vi "daq_intergration_v5.vi"() -> ()   [LabVIEW 2019]
uses:
  <vilib>/DAQmx/write.llb/DAQmx Write (Digital Bool 1Line 1Point).vi
  <vilib>/DAQmx/write.llb/DAQmx Write (Analog 1D DBL 1Chan NSamp).vi
  <vilib>/DAQmx/write.llb/DAQmx Write (Analog DBL 1Chan 1Samp).vi
  <vilib>/DAQmx/read.llb/DAQmx Read (Analog 1D Wfm NChan NSamp).vi
  <vilib>/DAQmx/create/channels.llb/DAQmx Create Channel (DO-Digital Output).vi
  <vilib>/DAQmx/miscellaneous.llb/DAQmx Fill In Error Info.vi
  <vilib>/DAQmx/create/channels.llb/DAQmx Create Channel (AI-Voltage-Basic).vi
  <vilib>/DAQmx/configure/timing.llb/DAQmx Timing (Sample Clock).vi
  <vilib>/DAQmx/configure/task.llb/DAQmx Configure Logging (TDMS).vi
  <vilib>/DAQmx/create/channels.llb/DAQmx Create Channel (AO-Voltage-Basic).vi
  <vilib>/measure/NI_MABase.lvlib
panel:
  in  "amplitude 3":dbl=2.5 caption="强刺激幅值" format="%0.2p"
  in  "强刺激频率":dbl=10.0 format="%#_13g"
  in  "低电平时间":dbl=15.0
  in  "高电平时间":dbl=10.0
  in  "physical channels 4":tag="Dev2/port0/line2" caption="行为视频输出通道"
  in  "行为视频":bool
  in  "刺激间隔下限(s)":dbl=3.0
  in  "刺激间隔上限":dbl=5.0
  in  "lines 2":tag="Dev2/port0/line1" caption="刺激事件通道"
  in  "frequency 2":dbl=10.0 caption="弱刺激频率" format="%0.2p"
  in  "amplitude 2":dbl=1.5 caption="弱刺激幅值" format="%0.2p"
  in  "amplitude":dbl=0.5 caption="超弱刺激幅值" format="%0.2p"
  in  "frequency":dbl=10.0 caption="超弱刺激频率" format="%0.2p"
  in  "physical channels 3":tag="Dev2/ao1" caption="胡须刺激通道"
  in  "胡须刺激":bool
  in  "data":dbl=2.0 caption="光源电压" format="%0.2f"
  in  "LED 光源":bool
  in  "physical channels 2":tag="Dev2/ao0" caption="LED通道"
  in  "lines":tag="Dev2/port0/line0" caption="事件通道"
  in  "?":bool
  in  "logging mode":i32(ring)=10231 caption="记录模式" items=["关"=10231, "记录"=15844, "记录并读取"=15842]
  in  "samples per channel":i32=1000 caption="每通道采样"
  in  "physical channels":tag="Dev2/ai0:3" caption="输入通道"
  in  "file path":path caption="文件路径"
  in  "停止":bool
  out "波形图":waveform(dbl)[](graph)
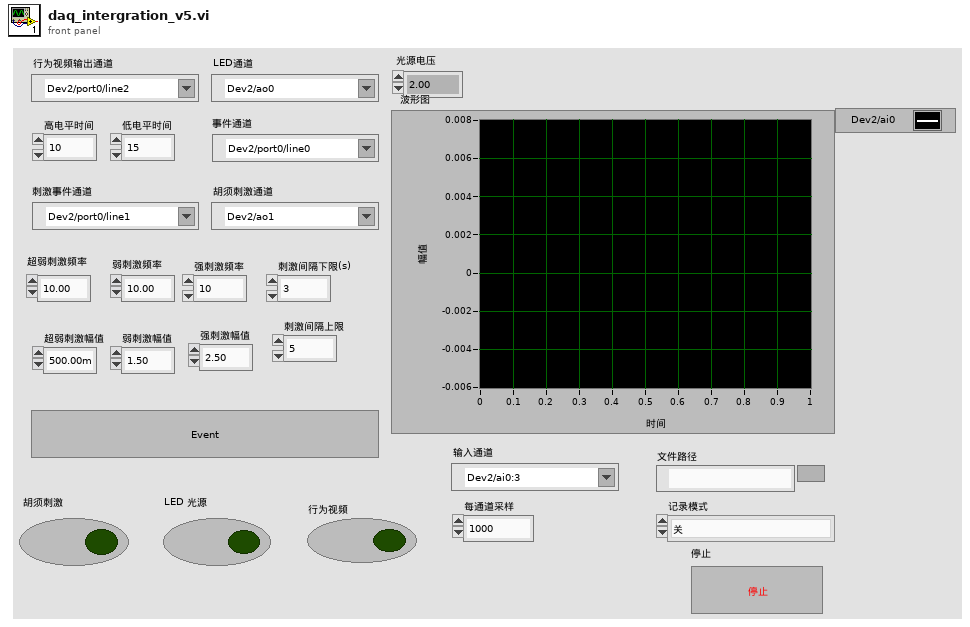
[diagram p1: front panel]
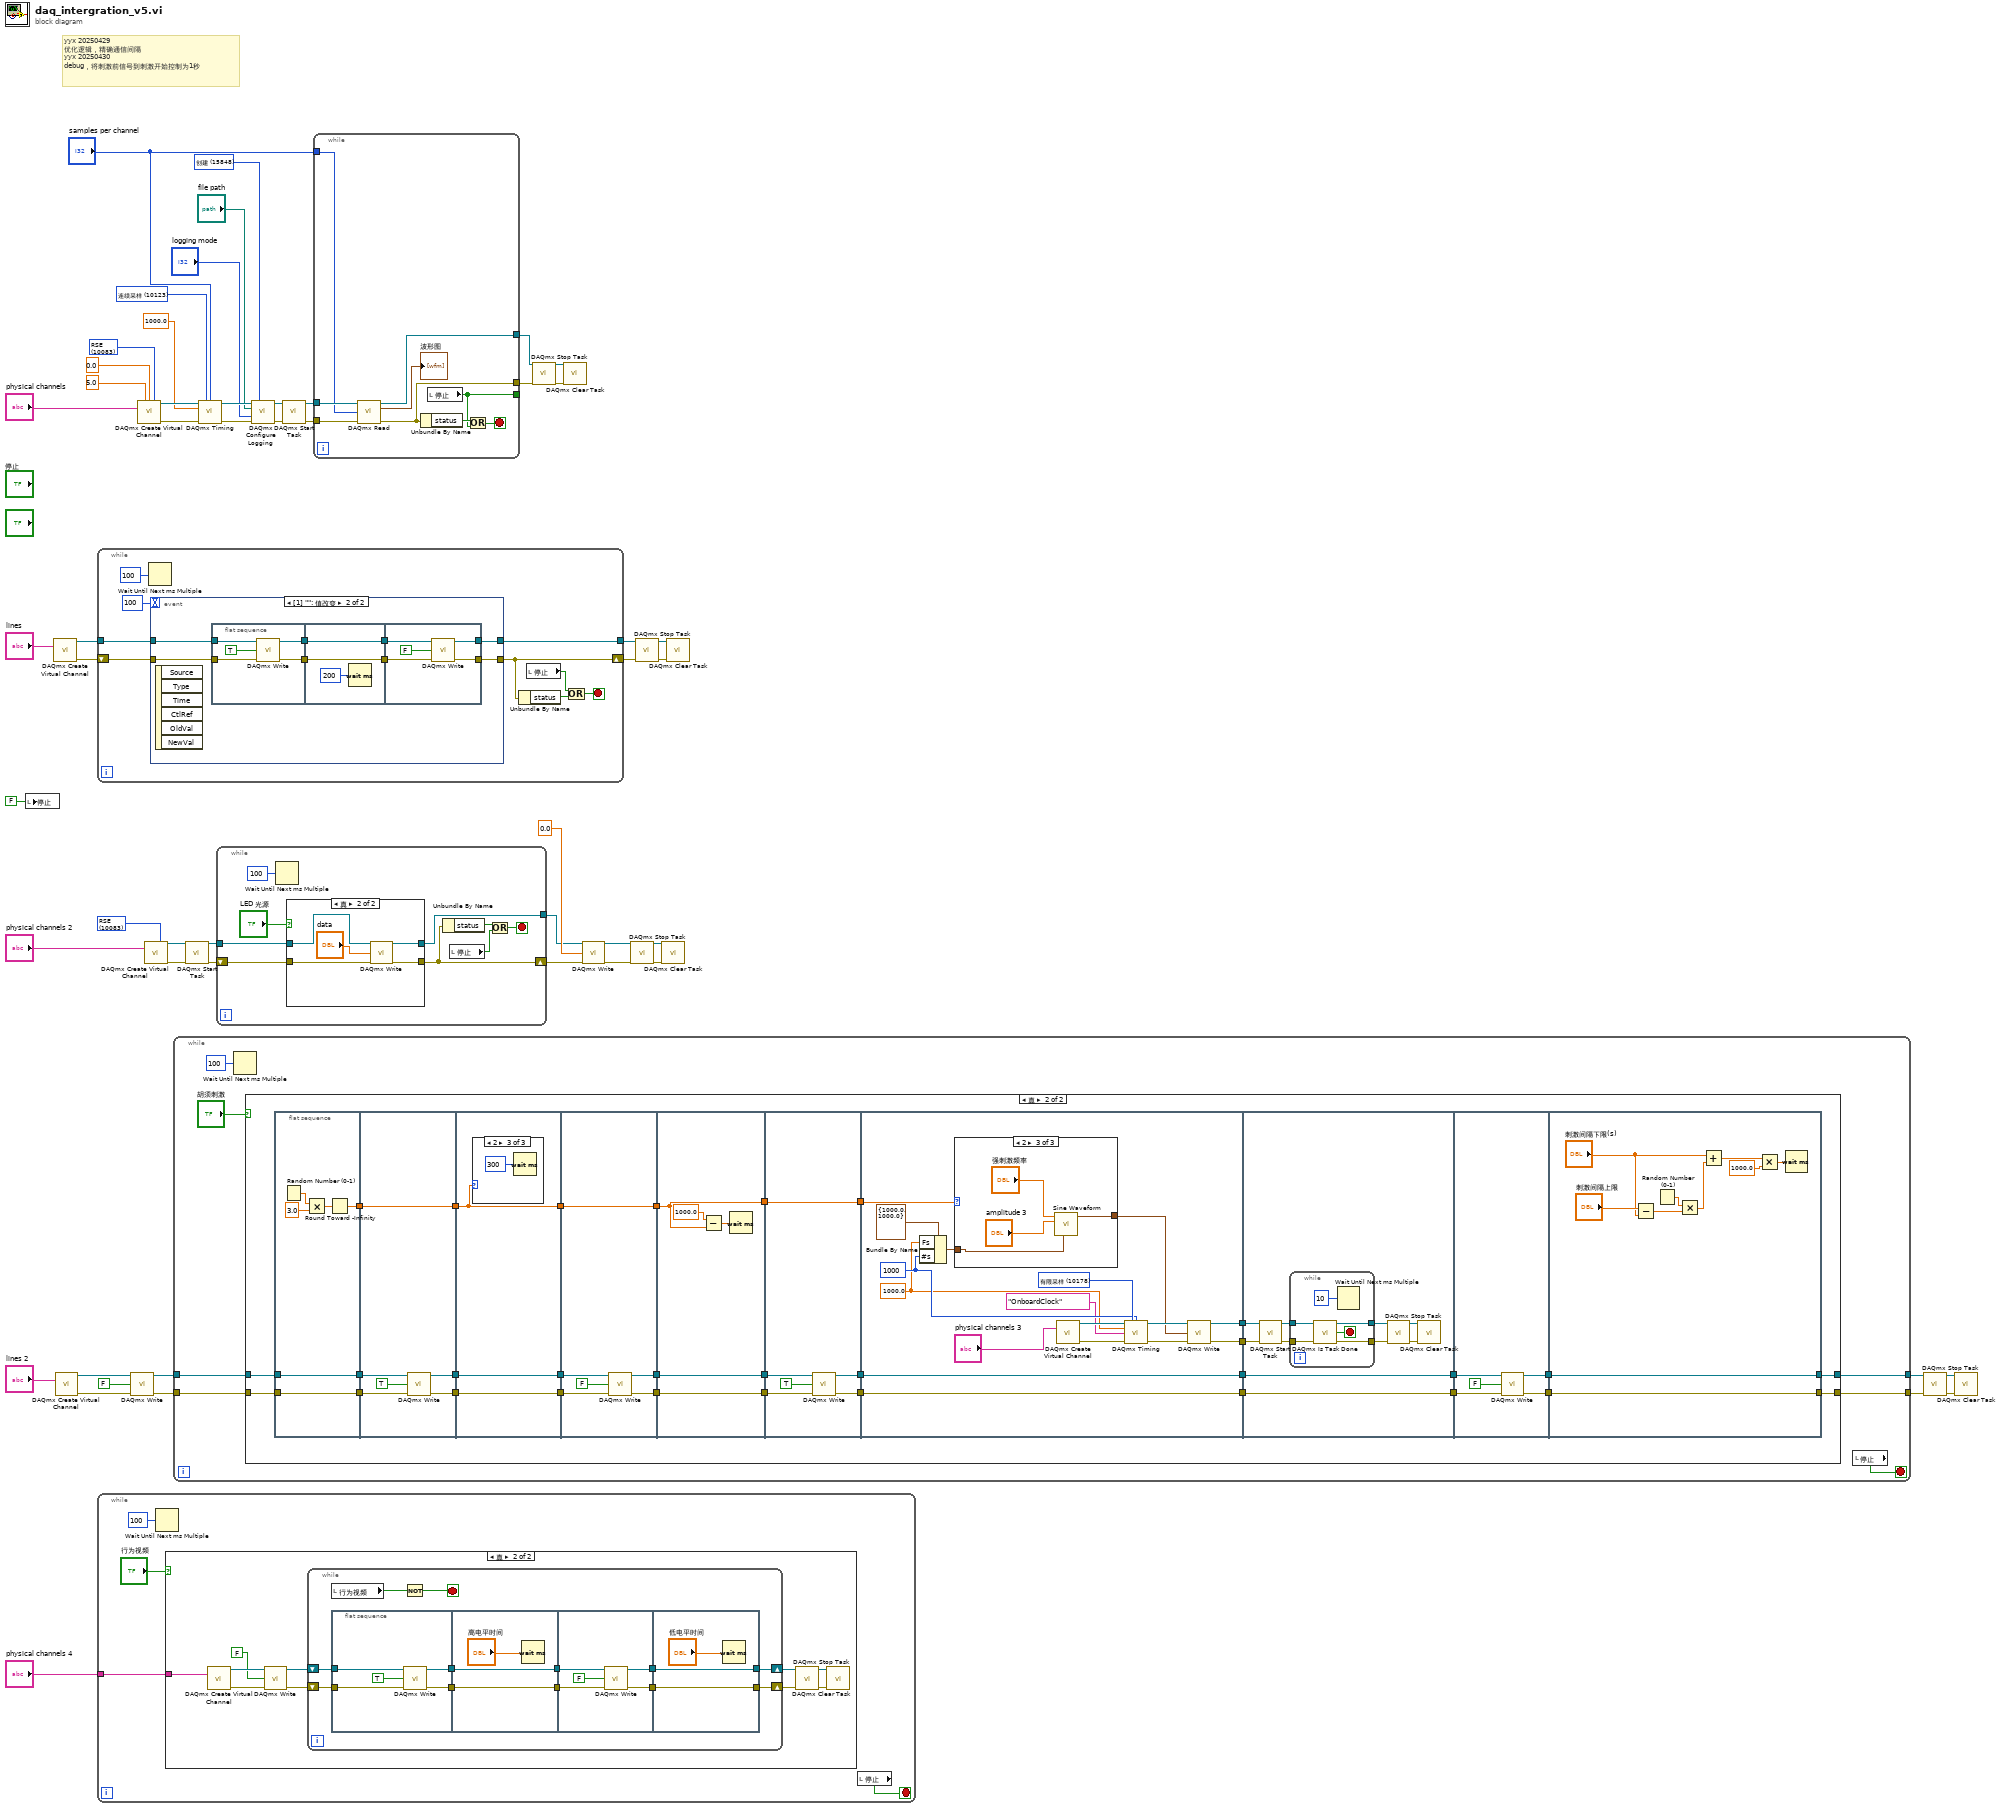
[diagram p0: block diagram]
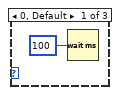
[diagram p4: hidden frame]
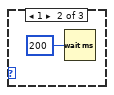
[diagram p5: hidden frame]
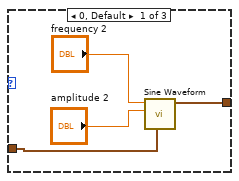
[diagram p6: hidden frame]
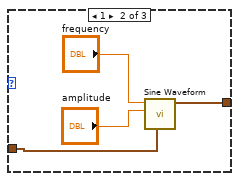
[diagram p7: hidden frame]
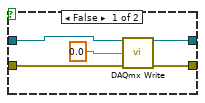
[diagram p8: hidden frame]
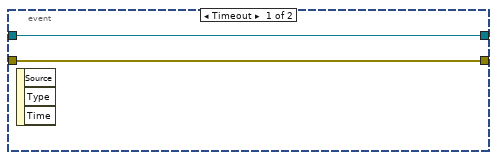
[diagram p9: hidden frame]
diagram:
  w14 = 10083 items=["默认"=-1, "RSE"=10083, "差分"=10106, "伪差分"=12529] ("output terminal configuration")
  w15 = 10083 items=["默认"=-1, "RSE"=10083, "NRSE"=10078, "差分"=10106, "伪差分"=12529] ("input terminal configuration")
  w45 = 15848 items=["打开"=10437, "打开或创建"=15846, "创建或替换"=15847, "创建"=15848] ("operation")
  w49 = 10123 items=["有限采样"=10178, "连续采样"=10123, "硬件定时单点"=12522] ("sample mode")
  # "yyx 20250429\n优化逻辑，精确通信间隔\nyyx 20250430\ndebug，将刺激前信号到刺激开始控制为1秒"
  n1 = local write "停止"(FALSE) -> ()
  n2 = call-poly <vilib>:"DAQmx Create Virtual Channel.vi"("lines"="lines") -> ("task out"=w31:refnum<k21>, "error out"=w30:errorcluster)  [unwired: 13 in]
  n3 = call-poly <vilib>:"DAQmx Create Virtual Channel.vi"("lines"="lines 2") -> ("task out"=w12:refnum<k21>, "error out"=w11:errorcluster)  [unwired: 13 in]
  n4 = while {
    shift-right: [w59] -> w28
    shift-left: w30 -> [w62]
    tunnel: w31 -> [w63]
    tunnel: [w61] -> w29
    stop <- w56 stop-if-true
    n5 = Wait Until Next ms Multiple(millisecond multiple=u32 100) -> ()  [unwired: 1 out]
    n6 = event shown="[1] \"\": 值改变" {
      selector: _ -> [_ _]
      dyn-events: _ -> [_ _]
      timeout: 100 -> [_ _]
      tunnel: w63 -> [w65 w73]
      tunnel: w62 -> [w64 w70]
      tunnel: [w65 w67] -> w61
      tunnel: [w64 w66] -> w59
      event Timeout {
        n7 = event-data() -> ()  [unwired: 1 in, 3 out]
      }
      event Value Change {
        n8 = event-data() -> ()  [unwired: 1 in, 6 out]
        n9 = flat-sequence {
          tunnel: w73 -> [w77]
          tunnel: [w76] -> w71
          tunnel: w70 -> [w75]
          tunnel: [w74] -> w68
          tunnel: [w80] -> w72
          tunnel: w71 -> [w80]
          tunnel: [w79] -> w69
          tunnel: w68 -> [w79]
          tunnel: w72 -> [w85]
          tunnel: w69 -> [w84]
          tunnel: [w83] -> w67
          tunnel: [w82] -> w66
          frame #0 {
            n10 = call-poly <vilib>:"DAQmx Write.vi"("task/channels in"=w77, "data"=TRUE, "error in"=w75) -> ("task out"=w76:refnum<k21>, "error out"=w74:errorcluster)  [unwired: 10 in, 1 out]
          }
          frame #1 {
            n11 = Wait (ms)(milliseconds to wait=u32 200 ("等待时间（毫秒）")) -> ()  [unwired: 1 out]
          }
          frame #2 {
            n12 = call-poly <vilib>:"DAQmx Write.vi"("task/channels in"=w85, "data"=FALSE, "error in"=w84) -> ("task out"=w83:refnum<k21>, "error out"=w82:errorcluster)  [unwired: 10 in, 1 out]
          }
        }
      }
    }
    n13 = Unbundle By Name(w59) -> ("status"=w58:bool)
    n14 = local read "停止"() -> (w57:bool)
    n15 = Or(x=w57, y=w58) -> (x .or. y?=w56:bool)
  }
  n16 = while {
    tunnel: "physical channels 4" -> [w90]
    stop <- w89 stop-if-true
    n17 = Wait Until Next ms Multiple(millisecond multiple=u32 100) -> ()  [unwired: 1 out]
    n18 = case shown="真" "行为视频" {
      tunnel: w90 -> [_ w100]
      frame False {
      }
      frame True {
        n19 = call-poly <vilib>:"DAQmx Create Virtual Channel.vi"("lines"=w100) -> ("task out"=w99:refnum<k21>, "error out"=w98:errorcluster)  [unwired: 13 in]
        n20 = call-poly <vilib>:"DAQmx Write.vi"("task/channels in"=w99, "data"=FALSE, "error in"=w98) -> ("task out"=w96:refnum<k21>, "error out"=w95:errorcluster)  [unwired: 10 in, 1 out]
        n21 = while {
          shift-right: [w110] -> w93
          shift-left: w96 -> [w112]
          shift-right: [w109] -> w92
          shift-left: w95 -> [w111]
          stop <- w107 stop-if-true
          n22 = local read "行为视频"() -> (w108:bool)
          n23 = flat-sequence {
            tunnel: w112 -> [w117]
            tunnel: w111 -> [w116]
            tunnel: [w114] -> w106
            tunnel: [w113] -> w104
            tunnel: w106 -> [w120]
            tunnel: [w120] -> w105
            tunnel: w104 -> [w119]
            tunnel: [w119] -> w103
            tunnel: w105 -> [w125]
            tunnel: w103 -> [w124]
            tunnel: [w123] -> w102
            tunnel: [w122] -> w101
            tunnel: [w127] -> w109
            tunnel: [w128] -> w110
            tunnel: w102 -> [w128]
            tunnel: w101 -> [w127]
            frame #0 {
              n24 = call-poly <vilib>:"DAQmx Write.vi"("task/channels in"=w117, "data"=TRUE, "error in"=w116) -> ("task out"=w114:refnum<k21>, "error out"=w113:errorcluster)  [unwired: 10 in, 1 out]
            }
            frame #1 {
              n25 = Wait (ms)(milliseconds to wait="高电平时间") -> ()  [unwired: 1 out]
            }
            frame #2 {
              n26 = call-poly <vilib>:"DAQmx Write.vi"("task/channels in"=w125, "data"=FALSE, "error in"=w124) -> ("task out"=w123:refnum<k21>, "error out"=w122:errorcluster)  [unwired: 10 in, 1 out]
            }
            frame #3 {
              n27 = Wait (ms)(milliseconds to wait="低电平时间") -> ()  [unwired: 1 out]
            }
          }
          n28 = Not(x=w108) -> (.not. x?=w107:bool)
        }
        n29 = call <vilib>:"DAQmx Stop Task.vi"("task/channels in"=w93, "error in"=w92) -> ("task out"=w94:refnum<k21>, "error out"=w91:errorcluster)  [unwired: 12 in]
        n30 = call <vilib>:"DAQmx Clear Task.vi"("task in"=w94, "error in"=w91) -> ()  [unwired: 13 in, 1 out]
      }
    }
    n31 = local read "停止"() -> (w89:bool)
  }
  n32 = call-poly <vilib>:"DAQmx Write.vi"("task/channels in"=w12, "data"=FALSE, "error in"=w11) -> ("task out"=w10:refnum<k21>, "error out"=w9:errorcluster)  [unwired: 10 in, 1 out]
  n33 = call-poly <vilib>:"DAQmx Create Virtual Channel.vi"("maximum value"=5.0, "minimum value"=0.0, "input terminal configuration"=w15, "physical channels"="physical channels") -> ("task out"=w51:refnum<k21>, "error out"=w50:errorcluster)  [unwired: 10 in]
  n34 = call-poly <vilib>:"DAQmx Create Virtual Channel.vi"("output terminal configuration"=w14, "physical channels"="physical channels 2") -> ("task out"=w26:refnum<k21>, "error out"=w25:errorcluster)  [unwired: 12 in]
  n35 = while {
    tunnel: w10 -> [w133]
    tunnel: w9 -> [w132]
    tunnel: [w131] -> w3
    tunnel: [w130] -> w2
    stop <- w134 stop-if-true
    n36 = Wait Until Next ms Multiple(millisecond multiple=u32 100) -> ()  [unwired: 1 out]
    n37 = case shown="真" "胡须刺激" {
      tunnel: w133 -> [w137 w167]
      tunnel: w132 -> [w136 w166]
      tunnel: [w137 w165] -> w131
      tunnel: [w136 w164] -> w130
      frame False {
      }
      frame True {
        n38 = flat-sequence {
          tunnel: w166 -> [w172]
          tunnel: w167 -> [w173]
          tunnel: [w173] -> w143
          tunnel: [w172] -> w142
          tunnel: [w168] -> w141
          tunnel: w143 -> [w177]
          tunnel: w142 -> [w175]
          tunnel: w141 -> [w179]
          tunnel: [w179] -> w140
          tunnel: [w176] -> w139
          tunnel: [w174] -> w138
          tunnel: [w182] -> w160
          tunnel: [w181] -> w159
          tunnel: [w180] -> w158
          tunnel: w140 -> [w182]
          tunnel: w139 -> [w181]
          tunnel: w138 -> [w180]
          tunnel: [w191] -> w163
          tunnel: [w187] -> w162
          tunnel: [w186] -> w161
          tunnel: w158 -> [w189]
          tunnel: w159 -> [w190]
          tunnel: w160 -> [w191]
          tunnel: w163 -> [w193]
          tunnel: [w193] -> w149
          tunnel: w162 -> [w196]
          tunnel: [w196] -> w147
          tunnel: w161 -> [w195]
          tunnel: [w195] -> w145
          tunnel: w149 -> [w202]
          tunnel: [w202] -> w148
          tunnel: w147 -> [w200]
          tunnel: [w199] -> w146
          tunnel: w145 -> [w198]
          tunnel: [w197] -> w144
          tunnel: w148 -> [w208]
          tunnel: [w207] -> w157
          tunnel: [w206] -> w156
          tunnel: [w205] -> w155
          tunnel: w146 -> [w205]
          tunnel: [w204] -> w154
          tunnel: w144 -> [w204]
          tunnel: [w241] -> w153
          tunnel: [w240] -> w152
          tunnel: w157 -> [w233]
          tunnel: w156 -> [w232]
          tunnel: w155 -> [w241]
          tunnel: w154 -> [w240]
          tunnel: w153 -> [w251]
          tunnel: w152 -> [w248]
          tunnel: [w250] -> w151
          tunnel: [w249] -> w150
          tunnel: [w254] -> w165
          tunnel: [w253] -> w164
          tunnel: w151 -> [w254]
          tunnel: w150 -> [w253]
          frame #0 {
            n39 = Random Number (0-1)() -> (number: 0 to 1=w170:dbl)
            n40 = Multiply(x=w170, y=3.0) -> (x*y=w171:dbl)
            n41 = Round Toward -Infinity(1:w171) -> (0:w168:dbl)
          }
          frame #1 {
            n42 = call-poly <vilib>:"DAQmx Write.vi"("task/channels in"=w177, "data"=TRUE, "error in"=w175) -> ("task out"=w176:refnum<k21>, "error out"=w174:errorcluster)  [unwired: 10 in, 1 out]
          }
          frame #2 {
            n43 = case shown="2" w182 {
              frame 0, Default {
                n44 = Wait (ms)(milliseconds to wait=u32 100 ("等待时间（毫秒）")) -> ()  [unwired: 1 out]
              }
              frame 1 {
                n45 = Wait (ms)(milliseconds to wait=u32 200 ("等待时间（毫秒）")) -> ()  [unwired: 1 out]
              }
              frame 2 {
                n46 = Wait (ms)(milliseconds to wait=u32 300 ("等待时间（毫秒）")) -> ()  [unwired: 1 out]
              }
            }
          }
          frame #3 {
            n47 = call-poly <vilib>:"DAQmx Write.vi"("task/channels in"=w190, "data"=FALSE, "error in"=w189) -> ("task out"=w187:refnum<k21>, "error out"=w186:errorcluster)  [unwired: 10 in, 1 out]
          }
          frame #4 {
            n48 = Subtract(x=1000.0, y=w193) -> (x-y=w192:dbl)
            n49 = Wait (ms)(milliseconds to wait=w192) -> ()  [unwired: 1 out]
          }
          frame #5 {
            n50 = call-poly <vilib>:"DAQmx Write.vi"("task/channels in"=w200, "data"=TRUE, "error in"=w198) -> ("task out"=w199:refnum<k21>, "error out"=w197:errorcluster)  [unwired: 10 in, 1 out]
          }
          frame #6 {
            w217 = 10178 items=["有限采样"=10178, "连续采样"=10123, "硬件定时单点"=12522] ("sample mode")
            w213 = 1000.0 ("rate")
            w214 = 1000 ("samples per channel")
            n51 = Bundle By Name(cluster=cluster{"Fs":dbl, "#s":dbl} {"Fs"=1000.0, "#s"=1000.0} ("sampling info"), "Fs"=w213, "#s"=w214) -> (w212:cluster{"Fs":dbl, "#s":dbl})
            n52 = case shown="2" w208 {
              tunnel: w212 -> [w223 w227 w231]
              tunnel: [w220 w224 w228] -> w209
              frame 0, Default {
                n53 = call <vilib>:"Sine Waveform.vi"("sampling info"=w223, "amplitude"="amplitude 2", "frequency"="frequency 2") -> ("signal out"=w220:waveform(dbl))  [unwired: 7 in, 1 out]
              }
              frame 1 {
                n54 = call <vilib>:"Sine Waveform.vi"("sampling info"=w227, "amplitude"="amplitude", "frequency"="frequency") -> ("signal out"=w224:waveform(dbl))  [unwired: 7 in, 1 out]
              }
              frame 2 {
                n55 = call <vilib>:"Sine Waveform.vi"("sampling info"=w231, "amplitude"="amplitude 3", "frequency"="强刺激频率") -> ("signal out"=w228:waveform(dbl))  [unwired: 7 in, 1 out]
              }
            }
            n56 = call-poly <vilib>:"DAQmx Create Virtual Channel.vi"("physical channels"="physical channels 3") -> ("task out"=w218:refnum<k21>, "error out"=w219:errorcluster)  [unwired: 13 in]
            n57 = call-poly <vilib>:"DAQmx Timing.vi"("task/channels in"=w218, "sample mode"=w217, "samples per channel"=w214, "rate"=w213, "source"=tag "OnboardClock", "error in"=w219) -> ("task out"=w211:refnum<k21>, "error out"=w210:errorcluster)  [unwired: 8 in]
            n58 = call-poly <vilib>:"DAQmx Write.vi"("task/channels in"=w211, "data"=w209, "error in"=w210) -> ("task out"=w207:refnum<k21>, "error out"=w206:errorcluster)  [unwired: 10 in, 1 out]
          }
          frame #7 {
            n59 = call <vilib>:"DAQmx Start Task.vi"("task/channels in"=w233, "error in"=w232) -> ("task out"=w234:refnum<k21>, "error out"=w235:errorcluster)  [unwired: 12 in]
            n60 = while {
              tunnel: w234 -> [w246]
              tunnel: [w245] -> w237
              tunnel: w235 -> [w244]
              tunnel: [w243] -> w236
              stop <- w247 stop-if-true
              n61 = call <vilib>:"DAQmx Is Task Done.vi"("task/channels in"=w246, "error in"=w244) -> ("task out"=w245:refnum<k21>, "task done?"=w247:bool, "error out"=w243:errorcluster)  [unwired: 11 in]
              n62 = Wait Until Next ms Multiple(millisecond multiple=u32 10) -> ()  [unwired: 1 out]
            }
            n63 = call <vilib>:"DAQmx Stop Task.vi"("task/channels in"=w237, "error in"=w236) -> ("task out"=w238:refnum<k21>, "error out"=w239:errorcluster)  [unwired: 12 in]
            n64 = call <vilib>:"DAQmx Clear Task.vi"("task in"=w238, "error in"=w239) -> ()  [unwired: 13 in, 1 out]
          }
          frame #8 {
            n65 = call-poly <vilib>:"DAQmx Write.vi"("task/channels in"=w251, "data"=FALSE, "error in"=w248) -> ("task out"=w250:refnum<k21>, "error out"=w249:errorcluster)  [unwired: 10 in, 1 out]
          }
          frame #9 {
            n66 = Subtract(x="刺激间隔上限", y="刺激间隔下限(s)") -> (x-y=w260:dbl)
            n67 = Random Number (0-1)() -> (number: 0 to 1=w262:dbl)
            n68 = Multiply(x=w262, y=w260) -> (x*y=w259:dbl)
            n69 = Add(x="刺激间隔下限(s)", y=w259) -> (x+y=w257:dbl)
            n70 = Multiply(x=w257, y=1000.0) -> (x*y=w255:dbl)
            n71 = Wait (ms)(milliseconds to wait=w255) -> ()  [unwired: 1 out]
          }
        }
      }
    }
    n72 = local read "停止"() -> (w134:bool)
  }
  n73 = call <vilib>:"DAQmx Start Task.vi"("task/channels in"=w26, "error in"=w25) -> ("task out"=w24:refnum<k21>, "error out"=w23:errorcluster)  [unwired: 12 in]
  n74 = call-poly <vilib>:"DAQmx Timing.vi"("task/channels in"=w51, "sample mode"=w49, "samples per channel"="samples per channel", "rate"=1000.0, "error in"=w50) -> ("task out"=w48:refnum<k21>, "error out"=w47:errorcluster)  [unwired: 9 in]
  n75 = while {
    tunnel: w24 -> [w270]
    tunnel: [w268] -> w21
    shift-right: [w264] -> w20
    shift-left: w23 -> [w269]
    stop <- w265 stop-if-true
    n76 = Wait Until Next ms Multiple(millisecond multiple=u32 100 ("毫秒倍数")) -> ()  [unwired: 1 out]
    n77 = case shown="真" "LED 光源" {
      tunnel: w270 -> [w276 w281]
      tunnel: w269 -> [w274 w280]
      tunnel: [w275 w278] -> w268
      tunnel: [w273 w277] -> w264
      frame False {
        n78 = call-poly <vilib>:"DAQmx Write.vi"("task/channels in"=w276, "data"=0.0, "error in"=w274) -> ("task out"=w275:refnum<k21>, "error out"=w273:errorcluster)  [unwired: 10 in, 1 out]
      }
      frame True {
        n79 = call-poly <vilib>:"DAQmx Write.vi"("task/channels in"=w281, "data"="data", "error in"=w280) -> ("task out"=w278:refnum<k21>, "error out"=w277:errorcluster)  [unwired: 10 in, 1 out]
      }
    }
    n80 = Unbundle By Name(w264) -> ("status"=w263:bool)
    n81 = local read "停止"() -> (w266:bool)
    n82 = Or(x=w263, y=w266) -> (x .or. y?=w265:bool)
  }
  n83 = call-poly <vilib>:"DAQmx Configure Logging.vi"("task/channels in"=w48, "operation"=w45, "file path"="file path", "logging mode"="logging mode", "error in"=w47) -> ("task out"=w44:refnum<k21>, "error out"=w43:errorcluster)  [unwired: 9 in]
  n84 = call <vilib>:"DAQmx Start Task.vi"("task/channels in"=w44, "error in"=w43) -> ("task out"=w42:refnum<k21>, "error out"=w41:errorcluster)  [unwired: 12 in]
  n85 = while {
    tunnel: w42 -> [w288]
    tunnel: w41 -> [w287]
    tunnel: "samples per channel" -> [w286]
    tunnel: [w284] -> w39
    tunnel: [w283] -> w37
    tunnel: [w282] -> _
    stop <- w285 stop-if-true
    n86 = call-poly <vilib>:"DAQmx Read.vi"("task/channels in"=w288, "number of samples per channel"=w286, "error in"=w287) -> ("task out"=w284:refnum<k21>, "data"=→"波形图":waveform(dbl)[], "error out"=w283:errorcluster)  [unwired: 10 in]
    n87 = Unbundle By Name(w283) -> ("status"=w290:bool)
    n88 = local read "停止"() -> (w282:bool)
    n89 = Or(x=w290, y=w282) -> (x .or. y?=w285:bool)
  }
  n90 = call <vilib>:"DAQmx Stop Task.vi"("task/channels in"=w39, "error in"=w37) -> ("task out"=w38:refnum<k21>, "error out"=w36:errorcluster)  [unwired: 12 in]
  n91 = call <vilib>:"DAQmx Clear Task.vi"("task in"=w38, "error in"=w36) -> ()  [unwired: 13 in, 1 out]
  n92 = call-poly <vilib>:"DAQmx Write.vi"("task/channels in"=w21, "data"=0.0, "error in"=w20) -> ("task out"=w17:refnum<k21>, "error out"=w16:errorcluster)  [unwired: 10 in, 1 out]
  n93 = call <vilib>:"DAQmx Stop Task.vi"("task/channels in"=w17, "error in"=w16) -> ("task out"=w19:refnum<k21>, "error out"=w18:errorcluster)  [unwired: 12 in]
  n94 = call <vilib>:"DAQmx Stop Task.vi"("task/channels in"=w29, "error in"=w28) -> ("task out"=w7:refnum<k21>, "error out"=w6:errorcluster)  [unwired: 12 in]
  n95 = call <vilib>:"DAQmx Clear Task.vi"("task in"=w19, "error in"=w18) -> ()  [unwired: 13 in, 1 out]
  n96 = call <vilib>:"DAQmx Clear Task.vi"("task in"=w7, "error in"=w6) -> ()  [unwired: 13 in, 1 out]
  n97 = call <vilib>:"DAQmx Stop Task.vi"("task/channels in"=w3, "error in"=w2) -> ("task out"=w5:refnum<k21>, "error out"=w4:errorcluster)  [unwired: 12 in]
  n98 = call <vilib>:"DAQmx Clear Task.vi"("task in"=w5, "error in"=w4) -> ()  [unwired: 13 in, 1 out]
